vi "gRPC Client Cache FGV Impl.vi"(8 "error in":errorcluster, 9 "unique id in":u64, 10 "action":T3, 11 "vi references in":T1) -> (0 "error out":errorcluster, 1 "unique id out":u64, 2 "grpc client id":T2, 3 "cluster id":string)   [LabVIEW 2020, in "Plug-In SDK Discovery V1.lvlib"]
uses:
  Plug-In SDK Discovery V1.lvlib
  TypeDefs/gRPC Client Cache FGV Action.ctl
  <vilib>/gRPC/LabVIEW gRPC Library/Shared/grpcId.ctl
  TypeDefs/gRPC Client Cache VI References.ctl
  <vilib>/gRPC/LabVIEW gRPC Library/grpc-lvsupport-release.lvlib
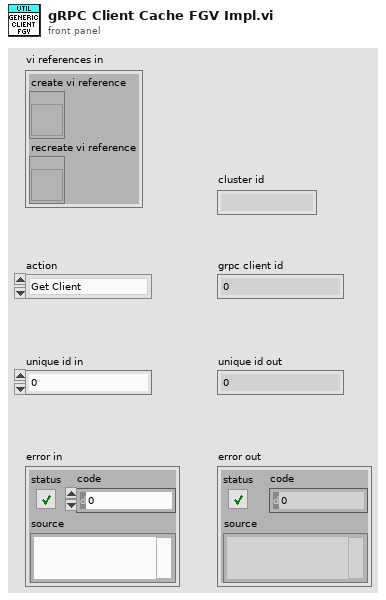
[diagram p1: front panel]
types:
  T1 = typedef "Plug-In SDK Discovery V1.lvlib/gRPC Client Cache VI References.ctl" = cluster{"create vi reference":refnum<vi>, "recreate vi reference":refnum<vi>}
  T2 = typedef "grpc-lvsupport-release.lvlib/grpcId.ctl" = u64
  T3 = typedef "Plug-In SDK Discovery V1.lvlib/gRPC Client Cache FGV Action.ctl" = enum16{"Get Client", "Recreate Client", "Destroy Client", "Update ClusterId"}
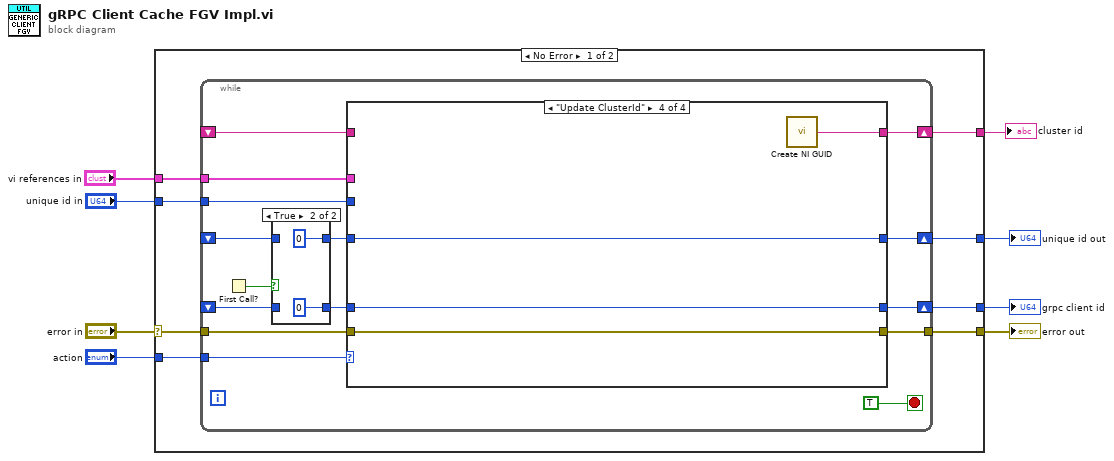
[diagram p0: block diagram]
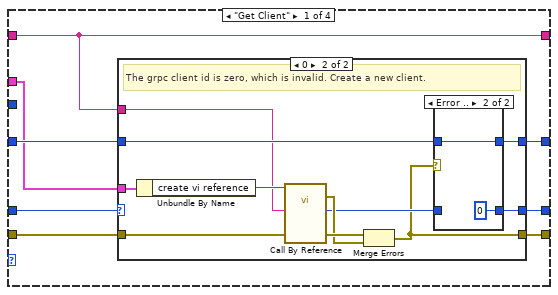
[diagram p3: hidden frame]
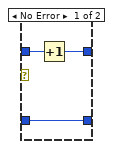
[diagram p5: hidden frame]
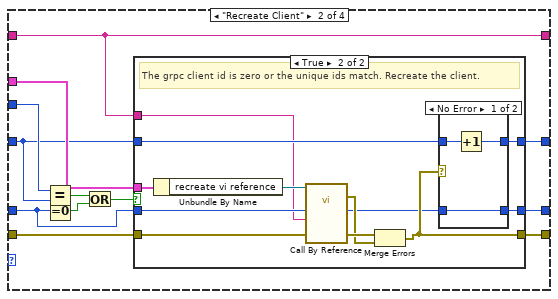
[diagram p6: hidden frame]
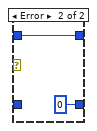
[diagram p8: hidden frame]
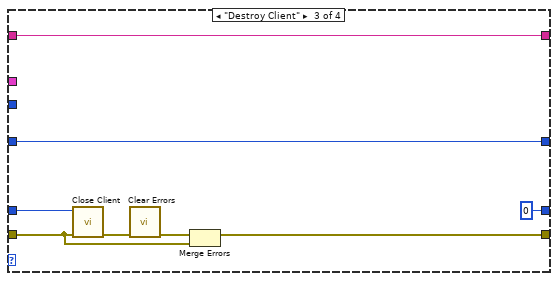
[diagram p9: hidden frame]
diagram:
  n1 = case shown="No Error" "error in" {
    selector: "error in" -> [w15 w107]
    tunnel: [w14 w107] -> w8
    tunnel: "action" -> [w16 _]
    tunnel: [w13 _] -> w7
    tunnel: [w12 _] -> w6
    tunnel: "unique id in" -> [w11 _]
    tunnel: "vi references in" -> [w10 _]
    tunnel: [w9 _] -> w1
    frame No Error {
      n2 = while {
        tunnel: w16 -> [w30]
        tunnel: w15 -> [w29]
        tunnel: [w28] -> w14
        shift-right: [w27] -> w13
        shift-left: _ -> [w25]
        shift-right: [w21] -> w12
        shift-left: _ -> [w23]
        tunnel: w11 -> [w20]
        tunnel: w10 -> [w19]
        shift-right: [w18] -> w9
        shift-left: _ -> [w17]
        stop <- TRUE stop-if-true
        n3 = First Call?() -> (First Call?: T/F=w26:bool)
        n4 = case shown="True" w26 {
          tunnel: w25 -> [w33 _]
          tunnel: [w33 T2 0 ("gRPC ID out")] -> w24
          tunnel: w23 -> [w32 _]
          tunnel: [w32 u64 0] -> w22
          frame False {
          }
          frame True {
          }
        }
        n5 = case shown="\"Update ClusterId\"" w30 {
          tunnel: w29 -> [w40 w73 w97 w103]
          tunnel: [w43 w74 w99 w103] -> w28
          tunnel: [w42 w71 T2 0 ("grpc client id out") w104] -> w27
          tunnel: w24 -> [w41 w64 w98 w104]
          tunnel: w22 -> [w39 w69 w95 w105]
          tunnel: [w38 w68 w95 w105] -> w21
          tunnel: w20 -> [_ w72 _ _]
          tunnel: w19 -> [w37 w70 _ _]
          tunnel: [w36 w63 w102 w106] -> w18
          tunnel: w17 -> [w36 w63 w102 _]
          frame "Get Client" {
            n6 = case shown="0" w41 {
              selector: w41 -> [w46 _]
              tunnel: w40 -> [w45 w56]
              tunnel: [w45 w48] -> w43
              tunnel: [w46 w51] -> w42
              tunnel: w39 -> [w44 w50]
              tunnel: [w44 w49] -> w38
              tunnel: w37 -> [_ w55]
              tunnel: w36 -> [_ w47]
              frame Default {
                # "The grpc client id is non-zero. As far as we know, it is valid, so return it."
              }
              frame 0 {
                # "The grpc client id is zero, which is invalid. Create a new client."
                n7 = Unbundle By Name(w55) -> ("create vi reference"=w57:refnum<vi>)
                n8 = call-by-ref "?"(reference=w57, "error in"=w56, "cluster id"=w47) -> (error out=w53:errorcluster, 0:"error out"=w54:errorcluster, "grpc client id"=w52:T2)  [unwired: 9 in, 1 out]
                n9 = Merge Errors(w54, w53) -> (w48:errorcluster)
                n10 = case shown="Error .." w48 {
                  tunnel: w50 -> [w60 w61]
                  tunnel: [w59 w61] -> w49
                  tunnel: w52 -> [w58 _]
                  tunnel: [w58 T2 0 ("grpc client id out")] -> w51
                  frame No Error {
                    n11 = Increment(x=w60) -> (x+1=w59:u64)
                  }
                  frame Error {
                  }
                }
              }
            }
          }
          frame "Recreate Client" {
            n12 = Equal?(x=w72, y=w69) -> (x = y?=w67:bool)
            n13 = Equal To 0?(x=w64) -> (x = 0?=w65:bool)
            n14 = Or(x=w67, y=w65) -> (x .or. y?=w66:bool)
            n15 = case shown="True" w66 {
              tunnel: w64 -> [w76 w87]
              tunnel: [w77 w83] -> w74
              tunnel: w73 -> [w77 w86]
              tunnel: [w76 w79] -> w71
              tunnel: w70 -> [_ w89]
              tunnel: w69 -> [w75 w82]
              tunnel: [w75 w81] -> w68
              tunnel: w63 -> [_ w78]
              frame False {
                # "The grpc client id is non-zero and the unique ids don't match. The client has already been recreated, so just return it."
              }
              frame True {
                # "The grpc client id is zero or the unique ids match. Recreate the client."
                n16 = Unbundle By Name(w89) -> ("recreate vi reference"=w88:refnum<vi>)
                n17 = call-by-ref "?"(reference=w88, "error in"=w86, "cluster id"=w78, "grpc client id in"=w87) -> (error out=w84:errorcluster, 0:"error out"=w85:errorcluster, "grpc client id out"=w80:T2)  [unwired: 8 in, 1 out]
                n18 = Merge Errors(w85, w84) -> (w83:errorcluster)
                n19 = case shown="No Error" w83 {
                  tunnel: w82 -> [w92 w94]
                  tunnel: [w91 w94] -> w81
                  tunnel: w80 -> [w90 _]
                  tunnel: [w90 T2 0 ("grpc client id out")] -> w79
                  frame No Error {
                    n20 = Increment(x=w92) -> (x+1=w91:u64)
                  }
                  frame Error {
                  }
                }
              }
            }
          }
          frame "Destroy Client" {
            n21 = call <vilib>:"Close Client.vi"("error in"=w97, "ClientID in"=w98) -> ("error out"=w96:errorcluster)  [unwired: 9 in]
            n22 = call <vilib>:"Clear Errors.vi"("error in (no error)"=w96) -> ("error out"=w100:errorcluster)  [unwired: 5 in, 1 out]
            n23 = Merge Errors(w100, w97) -> (w99:errorcluster)
          }
          frame "Update ClusterId" {
            n24 = call <vilib>:"Create NI GUID.vi"() -> ("NI GUID"=w106:string)
          }
        }
      }
    }
    frame Error {
    }
  }
  "error out" <- w8
  "grpc client id" <- w7
  "unique id out" <- w6
  "cluster id" <- w1
